vi "Pulse Gen Basic Scan.vi"(8 "error in (no error)":errorcluster, 10 "Pulse Generator.lvclass":refnum<class "Pulse Generator.lvclass">, 11 "Pulse Gen Basic Scan in":refnum<class "Pulse Gen Basic Scan.lvclass">) -> (0 "error out":errorcluster, 3 "Pulse Gen Basic Scan out":refnum<class "Pulse Gen Basic Scan.lvclass">)   [LabVIEW 2009, in "Pulse Gen Basic Scan.lvclass"]
uses:
  Pulse Gen Basic Scan.lvclass
  Instruments/Pulse Gen/Pulse Generator.lvclass
  Scanner/Scanner.lvclass
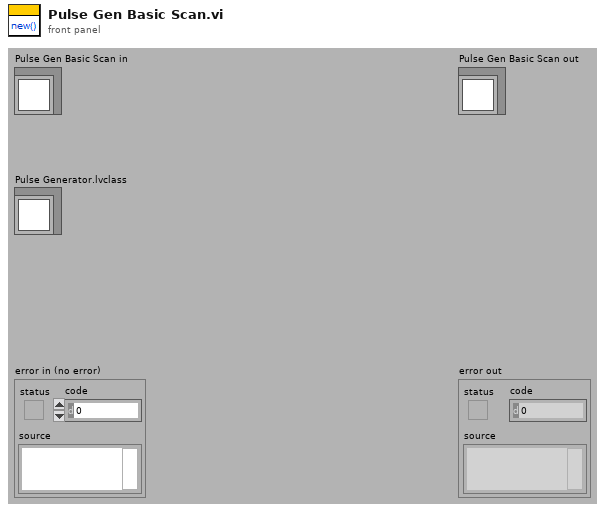
[diagram p1: front panel]
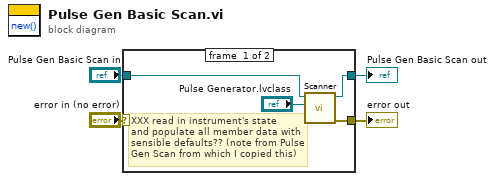
[diagram p0: block diagram]
diagram:
  n1 = case shown="No Error" "error in (no error)" {
    selector: "error in (no error)" -> [w6 w11]
    tunnel: [w5 w11] -> w3
    tunnel: [w7 w10] -> w1
    tunnel: "Pulse Gen Basic Scan in" -> [w8 w10]
    frame #0 {
      # "XXX read in instrument's state\nand populate all member data with\nsensible defaults?? (note from Pulse \nGen Scan from which I copied this)"
      n2 = call "Scanner.vi"("error in (no error)"=w6, "Scannable"="Pulse Generator.lvclass", "Scanner.lvclass in"=w8) -> ("error out"=w5:errorcluster, "Scanner.lvclass out"=w7:refnum<class "Pulse Gen Basic Scan.lvclass">)  [unwired: 1 in, 6 out]
    }
    frame #1 {
    }
  }
  "error out" <- w3
  "Pulse Gen Basic Scan out" <- w1
